vi "Create Map Entry Message.vi"(8 "error in (no error)":errorcluster, 10 "Map Definition":T5={"Message"="", "Definition"={"Name"="", "Number"=0, "Optional"=FALSE, "Repeated"=FALSE, "Type"={"Type"=enum."double", "Subtype"=""}, "Key Type"={"Type"=enum."double", "Subtype"=""}, "Value Type"={"Type"=enum."double", "Subtype"=""}}}, 11 "LV-Protoc in":refnum<class "LV-Protoc.lvclass">) -> (0 "error out":errorcluster, 2 "Message":T1, 3 "LV-Protoc out":refnum<class "LV-Protoc.lvclass">)   [LabVIEW 2020, in "LV-Protoc.lvlib" / "LV-Protoc.lvclass"]
uses:
  LV-Protoc.lvclass
  Map Definition.ctl
  LV-Proto/Field.ctl
  LV-Proto/Type.ctl
  LV-Proto/Proto Type.ctl
  LV-Proto/Message.ctl
  LV-Proto/LV-Proto.lvlib
  LV-Protoc.lvlib
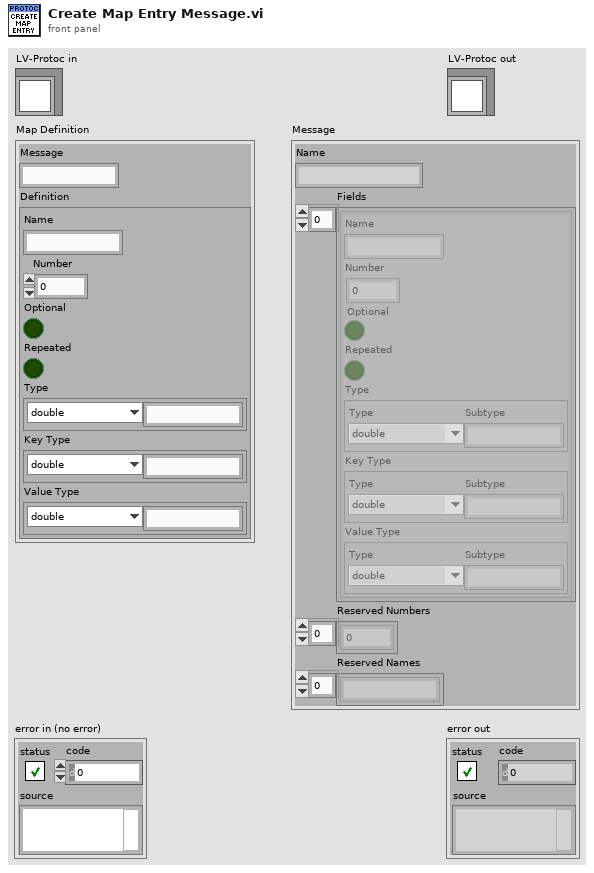
[diagram p1: front panel]
types:
  T1 = typedef "LV-Proto.lvlib/Message.ctl" = cluster{"Name":string, "Fields":T2[], "Reserved Numbers":u32[], "Reserved Names":string[]}
  T2 = typedef "LV-Proto.lvlib/Field.ctl" = cluster{"Name":string, "Number":u32, "Optional":bool, "Repeated":bool, "Type":T3, "Key Type":T3, "Value Type":T3}
  T3 = typedef "LV-Proto.lvlib/Type.ctl" = cluster{"Type":T4, "Subtype":string}
  T4 = typedef "LV-Proto.lvlib/Proto Type.ctl" = enum16{"UNKNOWN", "double", "float", "int32", "int64", "uint32", "uint64", "sint32", "sint64", "fixed32", "fixed64", "sfixed32", "sfixed64", "bool", "string", "bytes", "enum", "map", "message"}
  T5 = typedef "LV-Protoc.lvlib/Map Definition.ctl" = cluster{"Message":string, "Definition":T2}
  T6 = typedef "LV-Protoc.lvlib/Map Typenames.ctl" = cluster{"Entry":string, "Key":string, "Value":string}
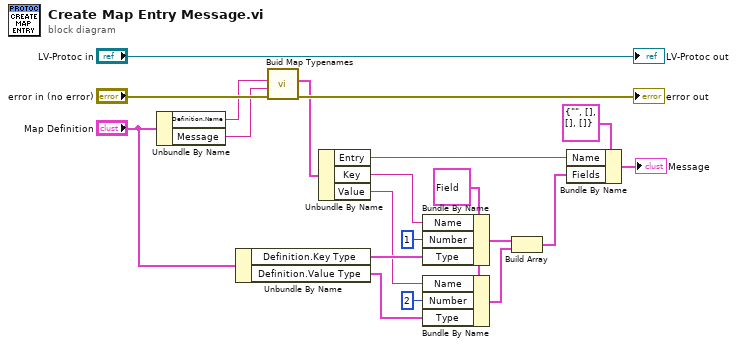
[diagram p0: block diagram]
diagram:
  w16 = T2 {"Name"="", "Number"=0, "Optional"=FALSE, "Repeated"=FALSE, "Type"={"Type"=enum."double", "Subtype"=""}, "Key Type"={"Type"=enum."double", "Subtype"=""}, "Value Type"={"Type"=enum."double", "Subtype"=""}} ("Field")
  n1 = Unbundle By Name("Map Definition") -> ("Definition.Name"=w4:string, "Message"=w2:string)
  n2 = Unbundle By Name("Map Definition") -> ("Definition.Key Type"=w19:T3, "Definition.Value Type"=w13:T3)
  n3 = call "Buid Map Typenames.vi"("error in (no error)"="error in (no error)", "Message Name"=w2, "Map Name"=w4) -> ("error out"=→"error out":errorcluster, "Map Typenames"=w6:T6)  [unwired: 7 in]
  n4 = Unbundle By Name(w6) -> ("Entry"=w1:string, "Key"=w17:string, "Value"=w15:string)
  n5 = Bundle By Name(cluster=w16, "Name"=w17, "Number"=u32 1, "Type"=w19) -> (w12:T2)
  n6 = Bundle By Name(cluster=w16, "Name"=w15, "Number"=u32 2, "Type"=w13) -> (w11:T2)
  n7 = Build Array(w12, w11) -> (w9:T2[])
  n8 = Bundle By Name(cluster=T1 {"Name"="", "Fields"=[], "Reserved Numbers"=[], "Reserved Names"=[]} ("Message"), "Name"=w1, "Fields"=w9) -> (→"Message":T1)
  "LV-Protoc out" <- "LV-Protoc in"
